vi "Secret Queue Name.vi"() -> (0 "name (unnamed)":string)   [LabVIEW 2017, in "Visualizer.lvlib"]
uses:
  Visualizer.lvlib
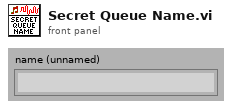
[diagram p1: front panel]
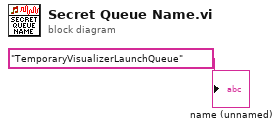
[diagram p0: block diagram]
diagram:
  "name (unnamed)" <- "TemporaryVisualizerLaunchQueue" ("name (unnamed)")
